vi "Max Read Single.vi"(8 "error in":errorcluster, 9 "Channel Index":i32=1, 11 "Max Temperature Limit in":refnum<class "Temperature Limit.lvclass">) -> (0 "error out":errorcluster, 1 "Changed or First Call?":bool, 2 "Current Setpoint":dbl, 3 "Max Temperature Limit out":refnum<class "Temperature Limit.lvclass">)   [LabVIEW 2023, in "Temperature Limit.lvclass"]
uses:
  Temperature Limit.lvclass
  Parents/Limit/Limit.lvclass
  Temperature Limit.lvclass/Temperature Limit.ctl
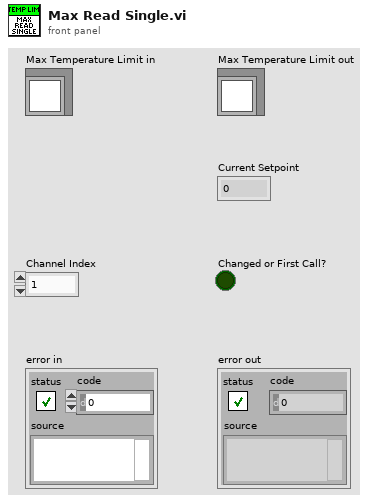
[diagram p1: front panel]
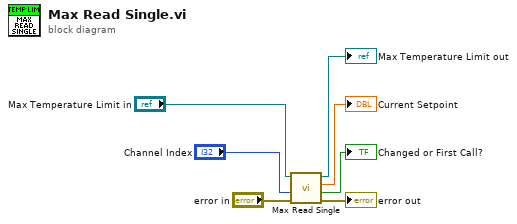
[diagram p0: block diagram]
diagram:
  n1 = call-parent "Max Read Single.vi"("error in"="error in", "Channel Index"="Channel Index", "Max Limit in"="Max Temperature Limit in") -> ("error out"=→"error out":errorcluster, "Changed or First Call?"=→"Changed or First Call?":bool, "Current Setpoint"=→"Current Setpoint":dbl, "Max Limit out"=→"Max Temperature Limit out":refnum<class "Temperature Limit.lvclass">)  [unwired: 5 in]
